vi "Add Token.vi"(7 "Token Type":T1, 8 "Length":i32=-1, 9 "Value Position":i32=-1, 10 "Next Position":i32=-1, 11 "Tokenizer In":T2) -> (3 "Tokenizer":T2)   [LabVIEW 2020, in "Stream.lvlib" / "URLPattern.lvclass"]
uses:
  URLPattern.lvclass
  Tokenizer.ctl
  Tokenize Policy.ctl
  Token.ctl
  Token Type.ctl
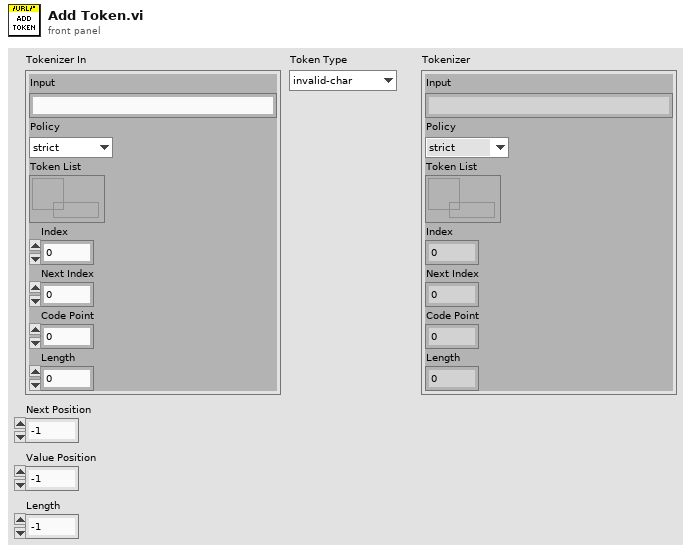
[diagram p1: front panel]
types:
  T1 = typedef "Stream.lvlib/URLPattern.lvclass/Token Type.ctl" = enum16{"invalid-char", "open", "close", "regexp", "name", "char", "escaped-char", "other-modifier", "asterisk", "end"}
  T2 = typedef "Stream.lvlib/URLPattern.lvclass/Tokenizer.ctl" = cluster{"Input":string, "Policy":T3, "Token List":refnum<queue>, "Index":i32, "Next Index":i32, "Code Point":u32, "Length":i32}
  T3 = typedef "Stream.lvlib/URLPattern.lvclass/Tokenize Policy.ctl" = enum16{"strict", "lenient"}
  T4 = typedef "Stream.lvlib/URLPattern.lvclass/Token.ctl" = cluster{"Type":T1, "Index":i32, "Value":string}
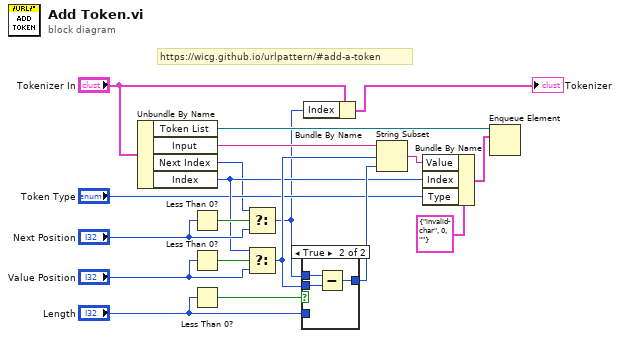
[diagram p0: block diagram]
diagram:
  # "https://wicg.github.io/urlpattern/#add-a-token"
  n1 = Unbundle By Name("Tokenizer In") -> ("Token List"=w6:refnum<queue>, "Input"=w18:string, "Next Index"=w2:i32, "Index"=w8:i32)
  n2 = Less Than 0?(x="Next Position") -> (x < 0?=w17:bool)
  n3 = Less Than 0?(x="Value Position") -> (x < 0?=w16:bool)
  n4 = Less Than 0?(x="Length") -> (x < 0?=w13:bool)
  n5 = Select(t=w2, s=w17, f="Next Position") -> (s? t:f=w1:i32)
  n6 = Select(t=w8, s=w16, f="Value Position") -> (s? t:f=w11:i32)
  n7 = case shown="True" w13 {
    tunnel: "Length" -> [w20 _]
    tunnel: w11 -> [_ w22]
    tunnel: w1 -> [_ w23]
    tunnel: [w20 w21] -> w10
    frame False {
    }
    frame True {
      n8 = Subtract(x=w23, y=w22) -> (x-y=w21:i32)
    }
  }
  n9 = Bundle By Name(cluster="Tokenizer In", "Index"=w1) -> (→"Tokenizer":T2)
  n10 = String Subset(string=w18, offset (0)=w11, length (rest)=w10) -> (substring=w9:string)
  n11 = Bundle By Name(cluster=T4 {"Type"=enum."invalid-char", "Index"=0, "Value"=""} ("Token"), "Value"=w9, "Index"=w8, "Type"="Token Type") -> (w5:T4)
  n12 = Enqueue Element(queue=w6, element=w5) -> ()  [unwired: 2 in, 3 out]
